vi "AVI-AVI2 Close all.vi"(8 "error in (no error)":errorcluster, 11 "AVI2 ref":T1[](array[typedef])) -> (0 "error out":errorcluster)   [LabVIEW 2020]
uses:
  <vilib>/vision/Avi.llb/IMAQ AVI2 Refnum.ctl
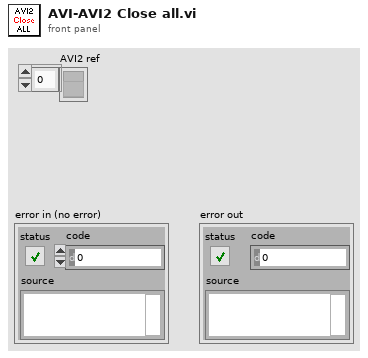
[diagram p1: front panel]
types:
  T1 = typedef "IMAQ AVI2 Refnum.ctl" = refnum<k20>
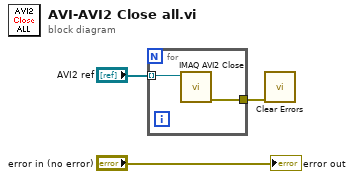
[diagram p0: block diagram]
diagram:
  n1 = for {
    tunnel: [w5] -> w3
    tunnel: "AVI2 ref" -> [w4] mode=indexing
    n2 = call "IMAQ AVI2 Close"("AVI Refnum"=w4) -> ("error out"=w5:errorcluster)  [unwired: 10 in]
  }
  n3 = call <vilib>:"Clear Errors.vi"("error in (no error)"=w3) -> ()  [unwired: 5 in, 2 out]
  "error out" <- "error in (no error)"
